vi "problem in clusters.vi"() -> ()   [LabVIEW 2011]
panel:
  out "Output":cluster{"Numeric":dbl, "Array":dbl[]}[](array[cluster])
  in  "Array":cluster{dbl, dbl[]}[](array[cluster])
  in  "SUBJECT NO":dbl
  in  "ROLL NO":dbl
  in  "NEW MARK":dbl
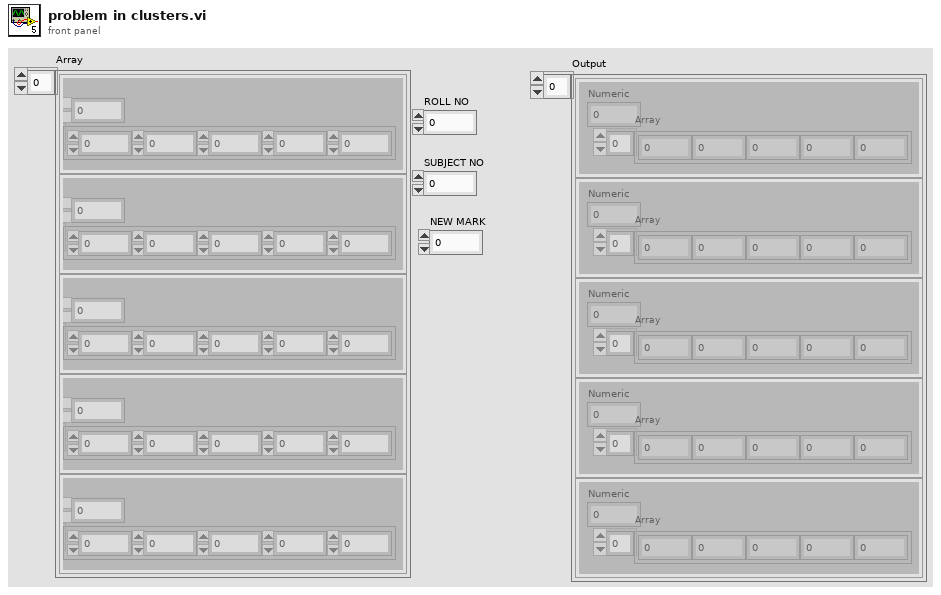
[diagram p1: front panel]
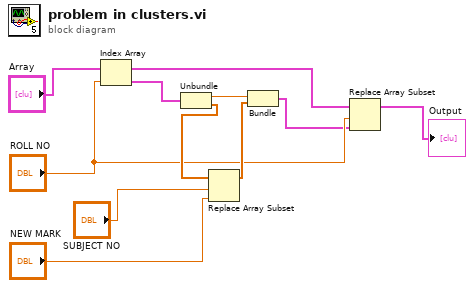
[diagram p0: block diagram]
diagram:
  n1 = Index Array(array="Array", index="ROLL NO") -> (element=w10:cluster{dbl, dbl[]})
  n2 = Unbundle(w10) -> (w9:dbl, w8:dbl[])
  n3 = Replace Array Subset(array=w8, new element="NEW MARK", index="SUBJECT NO") -> (w7:dbl[])
  n4 = Bundle(w9, w7) -> (w3:cluster{dbl, dbl[]})  [unwired: 1 in]
  n5 = Replace Array Subset(array="Array", new element=w3, index="ROLL NO") -> (→"Output":cluster{dbl, dbl[]}[])
